vi "cg_fid.vi"() -> ()   [LabVIEW 2011]
panel:
  in  "start Button":bool
  out "TCD":dbl(graph)
  out "FID":dbl(graph)
  in  "stop":bool
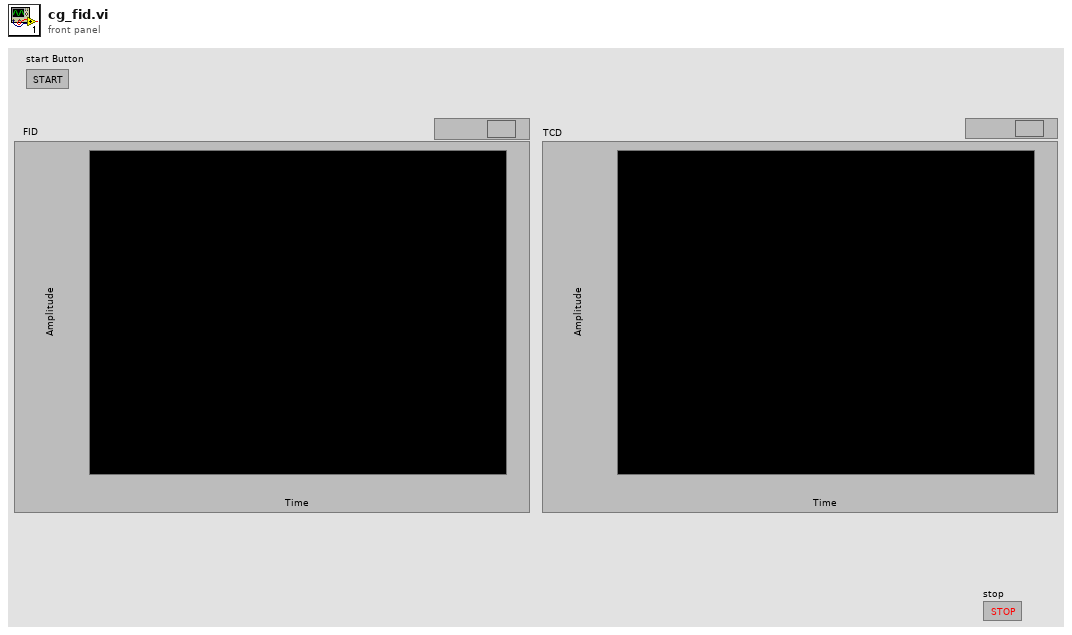
[diagram p1: front panel]
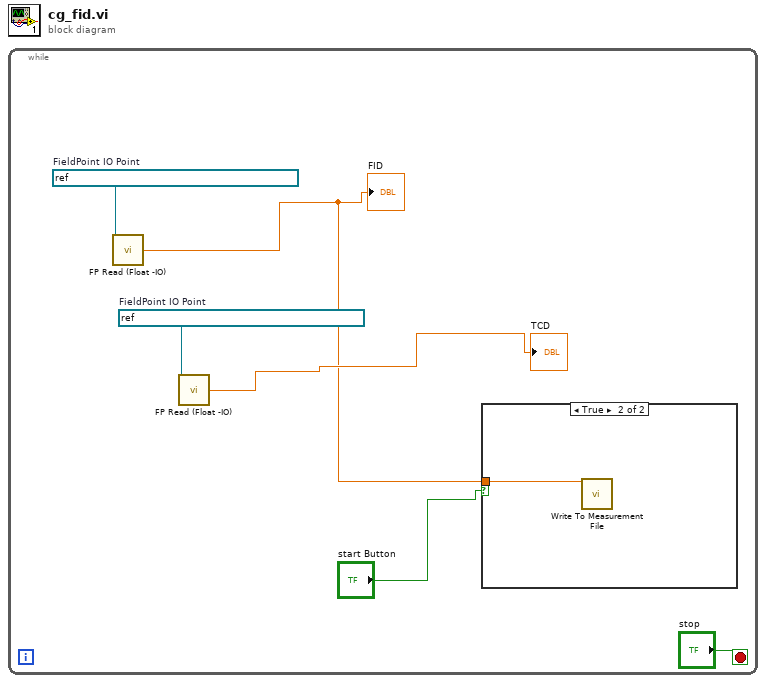
[diagram p0: block diagram]
diagram:
  n1 = while {
    stop <- "stop" stop-if-true
    w4 = refnum<k21> "FieldPoint\\cfp2220\\cFP-AI-110 @4\\Channel 2"  # FieldPoint IO Point
    w6 = refnum<k21> "FieldPoint\\cfp2220\\cFP-AI-110 @4\\Channel 0"  # FieldPoint IO Point
    n2 = call <vilib>:"FP Read (Float -IO).vi"("FieldPoint IO Point In"=w6) -> ("value"=w2:dbl)  [unwired: 11 in, 3 out]
    "FID" <- w2
    n3 = call <vilib>:"FP Read (Float -IO).vi"("FieldPoint IO Point In"=w4) -> ("value"=→"TCD":dbl)  [unwired: 11 in, 3 out]
    n4 = case shown="True" "start Button" {
      tunnel: w2 -> [_ w7]
      frame False {
      }
      frame True {
        n5 = call "Write To Measurement File"("Signals"=w7) -> ()  [unwired: 16 in, 3 out]
      }
    }
  }
